vi "2_Menu.vi"(0 "Disabled":T1(ring)) -> ()   [LabVIEW 2015]
panel:
  in  "Test 2":bool
  in  "manual":bool
  in  "Settings":bool
  in  "back":bool
  in  "Test":bool
  # "Developed by: VR Engineers"
  # "Contact: 9891971134"
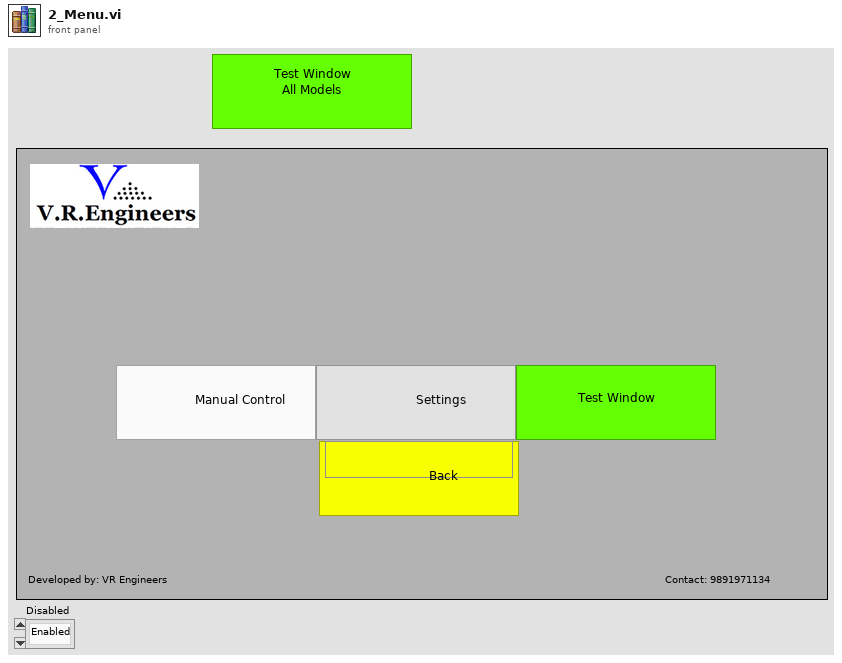
[diagram p1: front panel]
types:
  T1 = enum8{"Enabled", "Disabled", "Disabled and Grayed Out"}
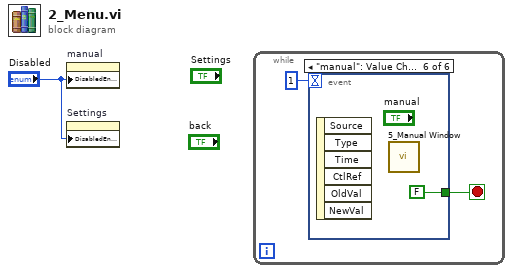
[diagram p0: block diagram]
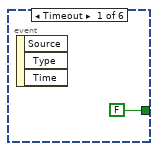
[diagram p2: hidden frame]
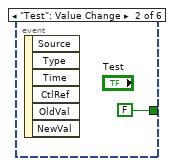
[diagram p3: hidden frame]
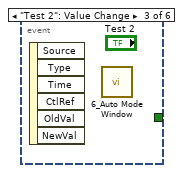
[diagram p4: hidden frame]
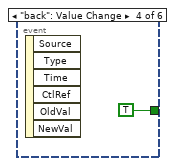
[diagram p5: hidden frame]
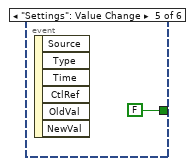
[diagram p6: hidden frame]
diagram:
  n1 = property on="manual" class="Bool"("DisabledEnum"="Disabled") -> ()  [unwired: 2 in, 2 out]
  n2 = property on="Settings" class="Bool"("DisabledEnum"="Disabled") -> ()  [unwired: 2 in, 2 out]
  n3 = while {
    stop <- w2 stop-if-true
    n4 = event shown="[5] \"manual\": Value Change" {
      selector: _ -> [_ _ _ _ _ _]
      dyn-events: _ -> [_ _ _ _ _ _]
      timeout: 1 -> [_ _ _ _ _ _]
      tunnel: [FALSE FALSE _ TRUE FALSE FALSE] -> w2
      event Timeout {
        n5 = event-data() -> ()  [unwired: 1 in, 3 out]
      }
      event "Test": Value Change {
        n6 = event-data() -> ()  [unwired: 1 in, 6 out]
      }
      event "Test 2": Value Change {
        n7 = event-data() -> ()  [unwired: 1 in, 6 out]
        n8 = call "6_Auto Mode Window.vi"() -> ()  [unwired: 12 in]
      }
      event "back": Value Change {
        n9 = event-data() -> ()  [unwired: 1 in, 6 out]
      }
      event "Settings": Value Change {
        n10 = event-data() -> ()  [unwired: 1 in, 6 out]
      }
      event "manual": Value Change {
        n11 = event-data() -> ()  [unwired: 1 in, 6 out]
        n12 = call "5_Manual Window.vi"() -> ()  [unwired: 12 in]
      }
    }
  }
